vi "Search Array for Multiple Instance_LV2012_NI Verified.vi"(9 "Array to Search":dbl[](array[numeric])=[5.0, 6.0, 4.0, 5.0, 8.0, 5.0, 9.0, 5.0, 6.0, 7.0, 5.0, 5.0], 10 "Number to find":dbl=5.0, 11 "Search Function/ Array Auto-Indexing":bool) -> (2 "Index Array":i32[](array[numeric]))   [LabVIEW 2017]
doc: "This VI will search an input 1D array for multiple instances of a single number and return an array containing the index values using 2 methods: Search 1D Array Function and Array Auto-Indexing"
panel:
  # "Overview: This VI will search an input 1D array for multiple instances of a single number and return an array containing the index values using 2 methods: Search 1D Array Function and Array Auto-Indexing\nRequirements: LabVIEW 2012 (or compatible)\nInstructions:\n1. Enter the number you want to find\n2. Click on the boolean control to choose the search method\n3. Run the VI"
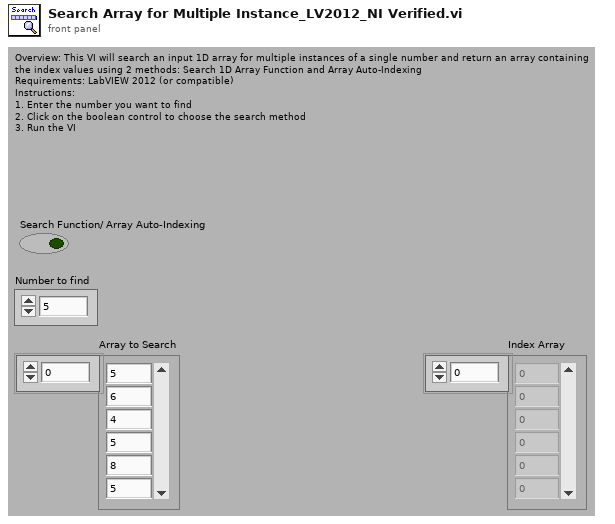
[diagram p1: front panel]
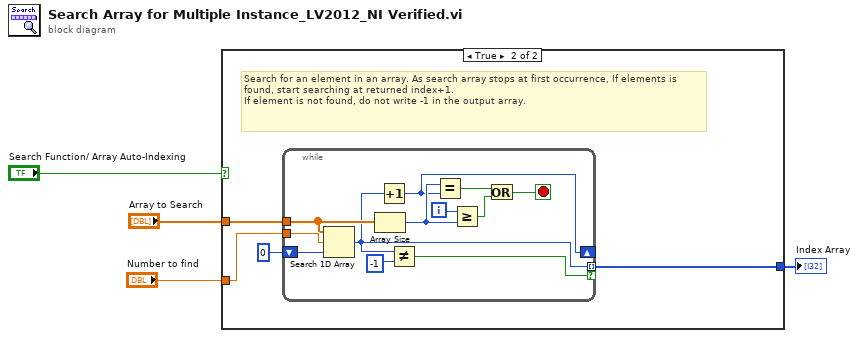
[diagram p0: block diagram]
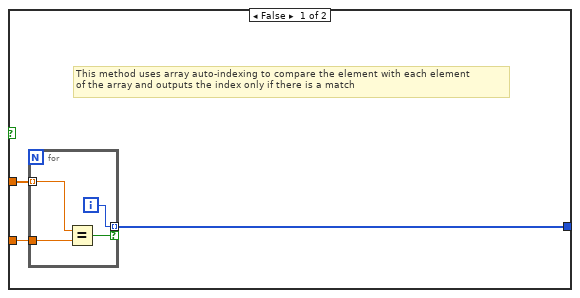
[diagram p2: hidden frame]
diagram:
  n1 = case shown="True" "Search Function/ Array Auto-Indexing" {
    tunnel: "Array to Search" -> [w7 w15]
    tunnel: "Number to find" -> [w6 w14]
    tunnel: [w5 w12] -> w1
    frame False {
      # "This method uses array auto-indexing to compare the element with each element \nof the array and outputs the index only if there is a match"
      n2 = for {
        tunnel: w7 -> [w11] mode=indexing
        tunnel: w6 -> [w10]
        tunnel: [w9] -> w5 mode=indexing if=w8
        i -> [w9]
        n3 = Equal?(x=w11, y=w10) -> (x = y?=w8:bool)
      }
    }
    frame True {
      # "Search for an element in an array. As search array stops at first occurrence, If elements is found, start searching at returned index+1.\nIf element is not found, do not write -1 in the output array."
      n4 = while {
        tunnel: w15 -> [w23]
        tunnel: w14 -> [w27]
        tunnel: [w16] -> w12 mode=indexing if=w25
        shift-right: [w18] -> _
        shift-left: 0 -> [w21]
        i -> [w24]
        stop <- w20 stop-if-true
        n5 = Search 1D Array(1D array=w23, element=w27, start index (0)=w21) -> (index of element=w16:i32)
        n6 = Array Size(array=w23) -> (size(s)=w19:i32)
        n7 = Increment(x=w16) -> (x+1=w18:i32)
        n8 = Not Equal?(x=w16, y=-1) -> (x != y?=w25:bool)
        n9 = Equal?(x=w19, y=w18) -> (x = y?=w17:bool)
        n10 = Greater Or Equal?(x=w24, y=w19) -> (x >= y?=w22:bool)
        n11 = Or(x=w17, y=w22) -> (x .or. y?=w20:bool)
      }
    }
  }
  "Index Array" <- w1
